vi "Homing Stage.vi"(8 "error in":errorcluster, 10 "Velocity":dbl, 11 ".NET Refnum in":refnum<k24>) -> (0 "error out":errorcluster, 3 ".NET Refnum out":refnum<k24>)   [LabVIEW 2013, in "ThorlabsLTS.lvclass"]
uses:
  ThorlabsLTS.lvclass
  C:/GEECS/Developers Version/builds/Device builds/ThorLabsLTS/Thorlabs.MotionControl.IntegratedStepperMotorsCLI.dll
  Thorlabs.MotionControl.IntegratedStepperMotorsCLI.dll
  C:/GEECS/Developers Version/builds/Device builds/ThorLabsLTS/Thorlabs.MotionControl.GenericMotorCLI.dll
  Thorlabs.MotionControl.GenericMotorCLI.dll
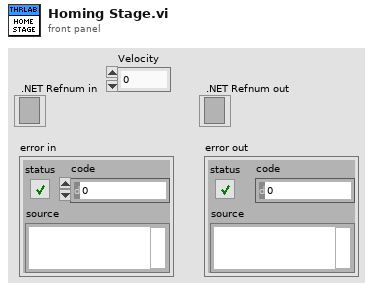
[diagram p1: front panel]
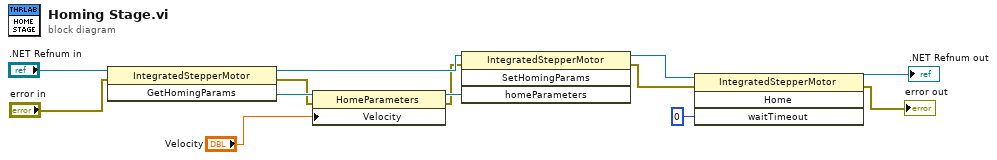
[diagram p0: block diagram]
diagram:
  n1 = invoke class="IntegratedStepperMotor" method="GetHomingParams"(reference=".NET Refnum in", error in="error in") -> (reference out=w7:refnum<k24>, error out=w2:errorcluster, "GetHomingParams"=w9:refnum<k24>)  [unwired: 1 in]
  n2 = property class="HomeParameters"(reference=w9, error in=w2, "Velocity"="Velocity") -> (reference out=w8:refnum<k24>, error out=w3:errorcluster)
  n3 = invoke class="IntegratedStepperMotor" method="SetHomingParams"(reference=w7, error in=w3, "homeParameters"=w8) -> (reference out=w4:refnum<k24>, error out=w5:errorcluster)  [unwired: 1 in, 2 out]
  n4 = invoke class="IntegratedStepperMotor" method="Home"(reference=w4, error in=w5, "waitTimeout"=0) -> (reference out=→".NET Refnum out":refnum<k24>, error out=→"error out":errorcluster)  [unwired: 1 in, 2 out]
